vi "Get Transfer Groups Pointer.vi"(11 "Framework Status in":refnum<class "Framework Status.lvclass">) -> (2 "transfer groups pointer":refnum<class "Status.lvclass">, 3 "Framework Status out":refnum<class "Framework Status.lvclass">)   [LabVIEW 2017, in "DSF Core.lvlib" / "Framework Status.lvclass"]
uses:
  Framework Status.lvclass
  Transfer Group Status/Status.lvclass
  Framework Status.lvclass/Framework Status.ctl
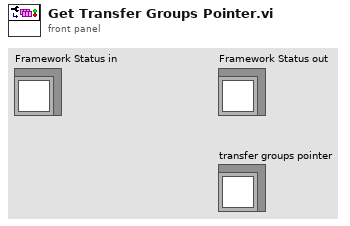
[diagram p1: front panel]
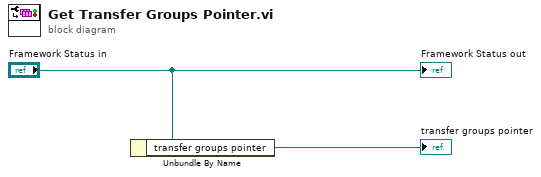
[diagram p0: block diagram]
diagram:
  n1 = Unbundle By Name("Framework Status in") -> ("transfer groups pointer"=→"transfer groups pointer":refnum<class "Status.lvclass">)
  "Framework Status out" <- "Framework Status in"
